vi "Read Lock-In Channel.vi"(7 "instance":i32, 8 "error in":errorcluster, 11 "lia host in":refnum<class "LIA Host Interface RT.lvclass">) -> (0 "error out":errorcluster, 2 "unscaled data":i64[][](array[numeric]), 3 "lia host out":refnum<class "LIA Host Interface RT.lvclass">)   [LabVIEW 2017, in "LIA Host Interface RT.lvclass"]
uses:
  LIA Host Interface RT.lvclass
  Properties/LockInQueues_GET.vi
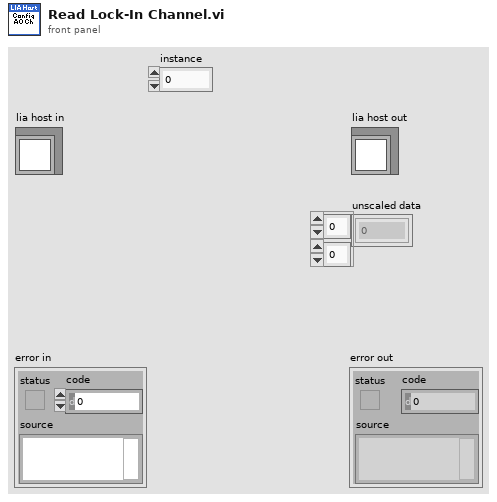
[diagram p1: front panel]
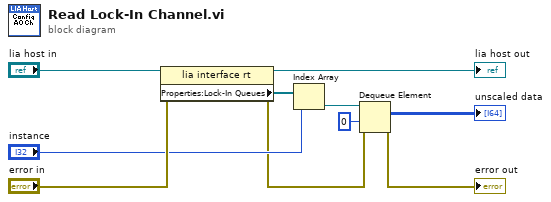
[diagram p0: block diagram]
diagram:
  n1 = property class="lia interface rt"(reference="lia host in", error in="error in") -> (reference out=→"lia host out":refnum<class "LIA Host Interface RT.lvclass">, error out=w2:errorcluster, "Properties:Lock-In Queues"=w7:refnum<queue>[])
  n2 = Index Array(array=w7, index="instance") -> (element=w5:refnum<queue>)
  n3 = Dequeue Element(queue=w5, timeout in ms (-1)=0, error in (no error)=w2) -> (element=→"unscaled data":i64[][], error out=→"error out":errorcluster)  [unwired: 2 out]
